vi "LcWebView_SimpleChart_Example.vi"() -> ()   [LabVIEW 2018, in "LcWebView.lvclass"]
doc: "Inject javascript arguments"
uses:
  LcWebView.lvclass
  D:/GitProjects/Public/GitHub/LcWebView/data/Microsoft.Web.WebView2.WinForms.dll
  data/Microsoft.Web.WebView2.WinForms.dll
panel:
  out "BrowserProcessId":u32
  out "Status Message":string
  in  "stop":bool
  in  "Web":refnum<k24>(container)
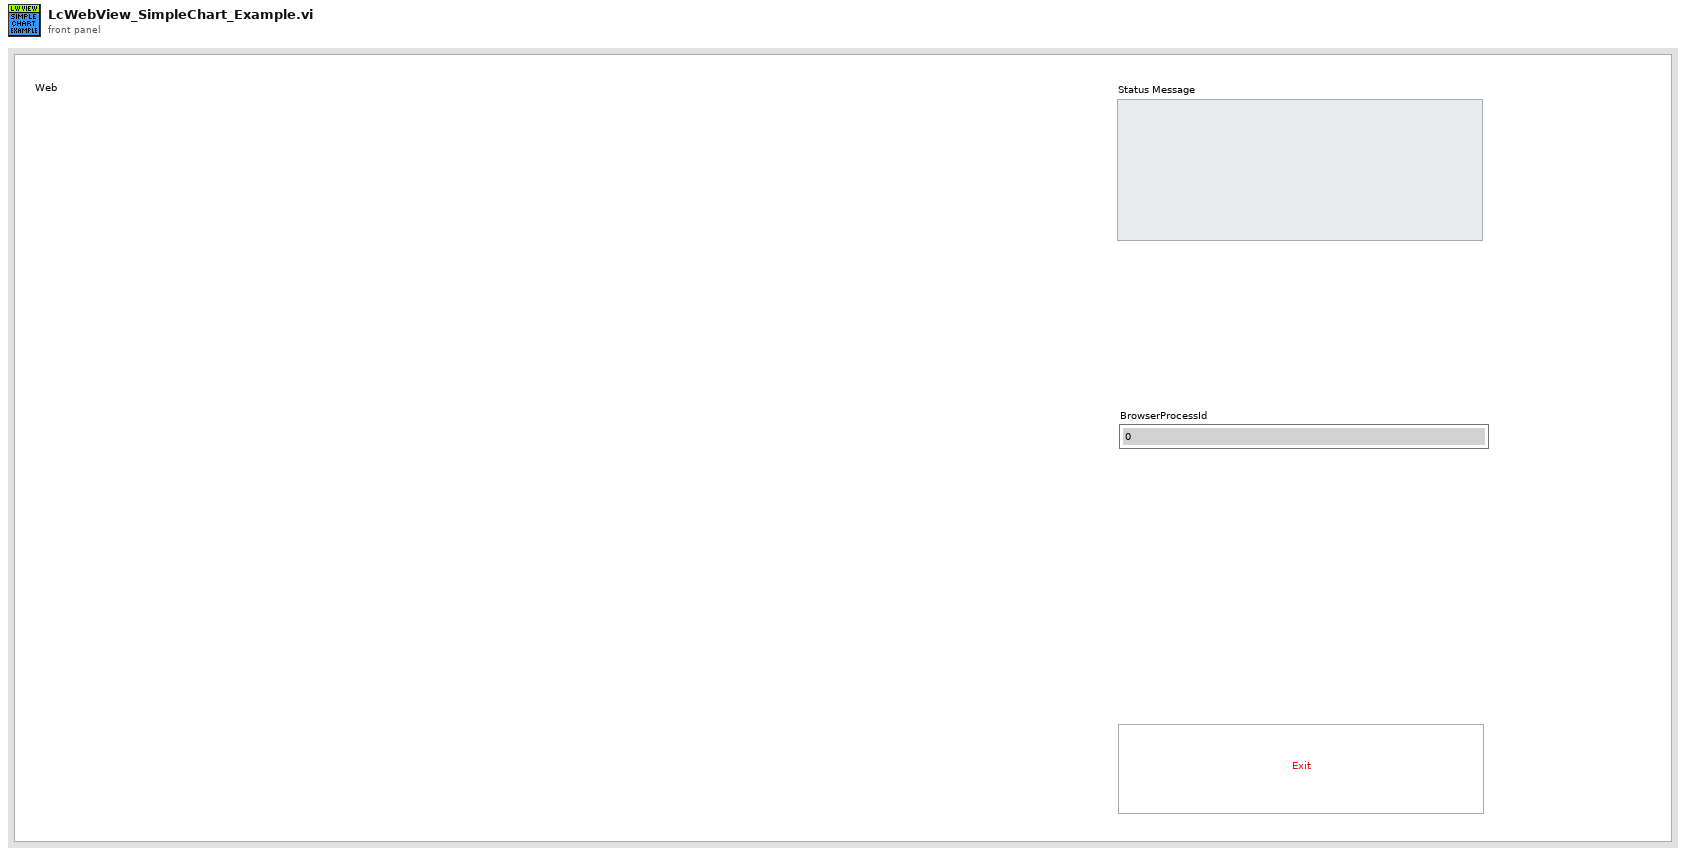
[diagram p1: front panel]
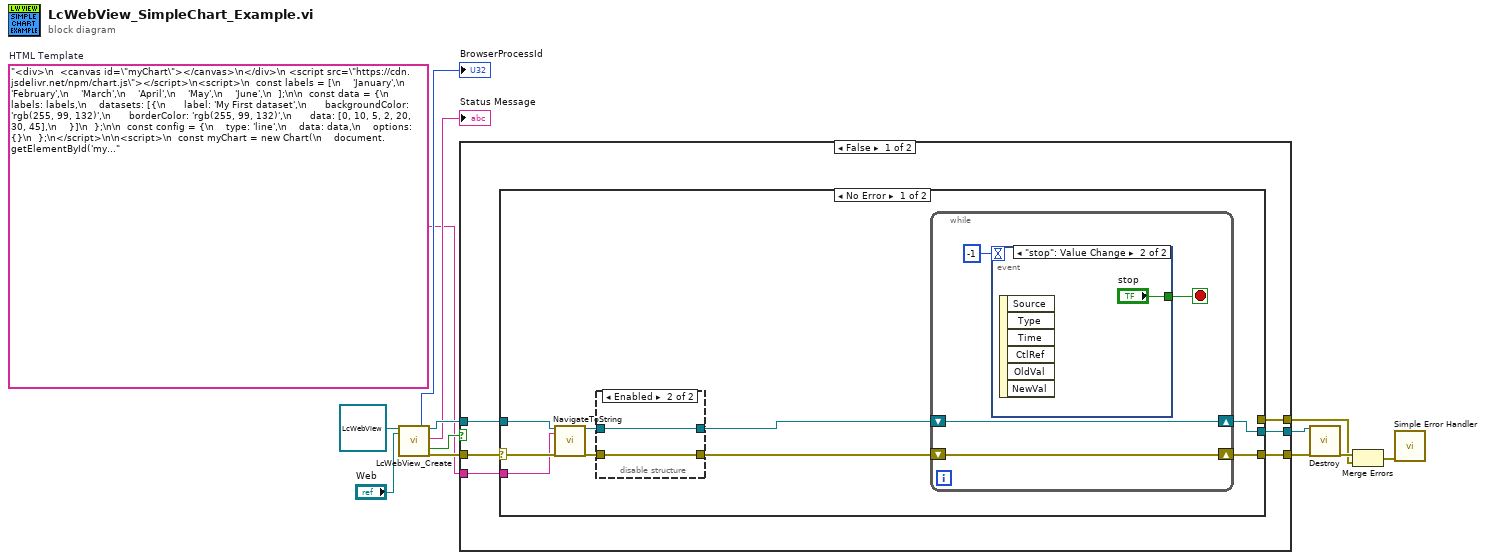
[diagram p0: block diagram]
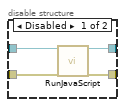
[diagram p2: hidden frame]
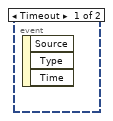
[diagram p3: hidden frame]
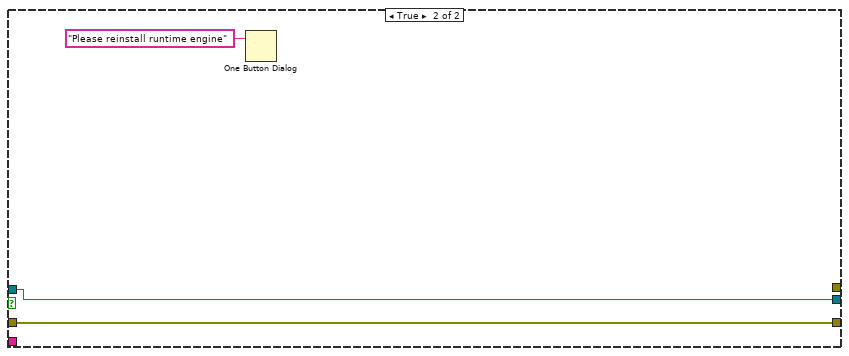
[diagram p5: hidden frame]
diagram:
  w2 = "<div>\n  <canvas id=\"myChart\"></canvas>\n</div>\n <script src=\"https://cdn.jsdelivr.net/npm/chart.js\"></script>\n<script>\n  const labels = [\n    'January',\n    'February',\n    'March',\n    'April',\n    'May',\n    'June',\n  ];\n\n  const data = {\n    labels: labels,\n    datasets: [{\n      label: 'My First dataset',\n      backgroundColor: 'rgb(255, 99, 132)',\n      borderColor: 'rgb(255, 99, 132)',\n      data: [0, 10, 5, 2, 20, 30, 45],\n    }]\n  };\n\n  const config = {\n    type: 'line',\n    data: data,\n    options: {}\n  };\n</script>\n\n<script>\n  const myChart = new Chart(\n    document.getElementById('myChart'),\n    config\n  );\n</script>"  # HTML Template
  n1 = call "LcWebView_Create.vi"("reference in"=refnum<class "LcWebView.lvclass"> refnum, "Webview container"="Web") -> ("BrowserProcessId"=→"BrowserProcessId":u32, "reference out"=w11:refnum<class "LcWebView.lvclass">, "Status Message"=→"Status Message":string, "Reinstall Runtime"=w4:bool, "Error Out"=w10:errorcluster)  [unwired: 10 in, 3 out]
  n2 = case shown="False" w4 {
    tunnel: w11 -> [w19 w44]
    tunnel: w10 -> [w18 w43]
    tunnel: [w17 w44] -> w9
    tunnel: [w15 w43] -> w8
    tunnel: [w16 _] -> w5
    tunnel: w2 -> [w14 _]
    frame False {
      n3 = case shown="No Error" w18 {
        selector: w18 -> [w26 w40]
        tunnel: w19 -> [w27 w41]
        tunnel: [w25 w41] -> w17
        tunnel: [w28 _] -> w15
        tunnel: [_ w40] -> w16
        tunnel: w14 -> [w23 _]
        frame No Error {
          n4 = call-dynamic "NavigateToString.vi"("reference in"=w27, "HTML Content"=w23, "Error In"=w26) -> ("reference out"=w24:refnum<class "LcWebView.lvclass">, "Error Out"=w22:errorcluster)  [unwired: 14 in, 1 out]
          n5 = disable-structure shown="Enabled" {
            disable-tunnel: [w32 w34] -> w21
            disable-tunnel: [w31 w33] -> w20
            disable-tunnel: w24 -> [w30 w34]
            disable-tunnel: w22 -> [w29 w33]
            frame Disabled {
              n6 = call-dynamic "RunJavaScript.vi"("reference in"=w30, "Error In"=w29) -> ("reference out"=w32:refnum<class "LcWebView.lvclass">, "Error Out"=w31:errorcluster)  [unwired: 14 in, 2 out]
            }
            frame Enabled {
            }
          }
          n7 = while {
            shift-right: [w38] -> w25
            shift-left: w21 -> [w38]
            shift-right: [w37] -> w28
            shift-left: w20 -> [w37]
            stop <- w35 stop-if-true
            n8 = event shown="[1] \"stop\": Value Change" {
              selector: _ -> [_ _]
              dyn-events: _ -> [_ _]
              timeout: -1 -> [_ _]
              tunnel: [_ "stop"] -> w35
              event Timeout {
                n9 = event-data() -> ()  [unwired: 1 in, 3 out]
              }
              event "stop": Value Change {
                n10 = event-data() -> ()  [unwired: 1 in, 6 out]
              }
            }
          }
        }
        frame Error {
        }
      }
    }
    frame True {
      n11 = One Button Dialog(message="Please reinstall runtime engine") -> ()  [unwired: 1 in, 1 out]
    }
  }
  n12 = call-dynamic "Destroy.vi"("reference in"=w9, "Error In"=w8) -> ("Error Out"=w7:errorcluster)  [unwired: 16 in, 1 out]
  n13 = Merge Errors(w7, w5) -> (w1:errorcluster)
  n14 = call <vilib>:"Simple Error Handler.vi"("error in (no error)"=w1) -> ()  [unwired: 4 in, 5 out]
